vi "AddDropletDBtoDBarrayAndDisplayInGraph.vi"(8 "error in (no error)":errorcluster, 11 "Queue In":refnum<queue>) -> (0 "error out":errorcluster, 3 "Queue Out":refnum<queue>)   [LabVIEW 2013]
doc: "Use this template to build a VI to use as a subVI."
uses:
  TypeDef/DisplayQueue.ctl
  TypeDef/DisplayEnum.ctl
  DB/DbEnum.ctl
  DB/ArrayofDropletsDBEnum.ctl
panel:
  # "Add droplet database to database array\nand update the normalized droplet graph \nas a function of temperature"
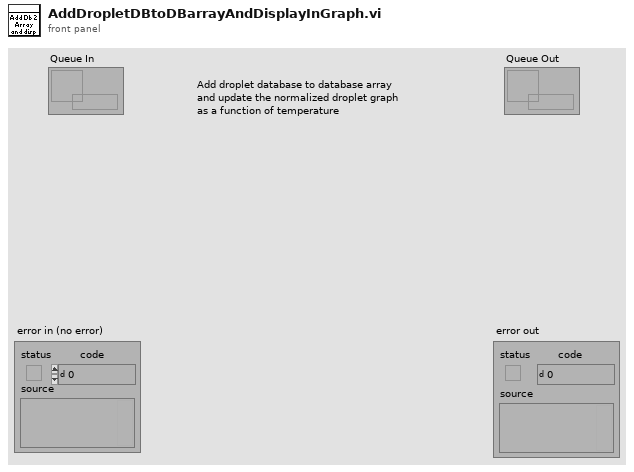
[diagram p1: front panel]
types:
  T1 = typedef "ArrayofDropletsDBEnum.ctl" = enum16{"AnalyzeDropletDBs", "PrepareDBforSave", "GetDBtoListBox", "UpdateDBtoListBox", "AddDBtoListBox", "AddDropletDB", "InitArrayOfDropletDB"}
  T2 = typedef "DisplayEnum.ctl" = enum16{"Stop Display", "Update Display", "Update Multiple Files Display", "Center Image", "Update Configuration Display", "Init Display"}
  T3 = typedef "DbEnum.ctl" = enum16{"RemoveOneDroplet", "AddOneDroplet", "Write DropletDB", "Init", "Insert Detection Result Data", "Insert Grey Level Result", "Insert Baseline Results", "AddFreezeImagesAtCertainDroplet", "UpdateIncludeDroplet", "Insert Freeze Analysis Results", "GetDropDB", "GetNoFreezedDroplets", "GetGreyLevelAndDiff", "GetGreyLevelatIndexTime", "GetDropletsBoundingBox", "GetDropletsDiameter"}
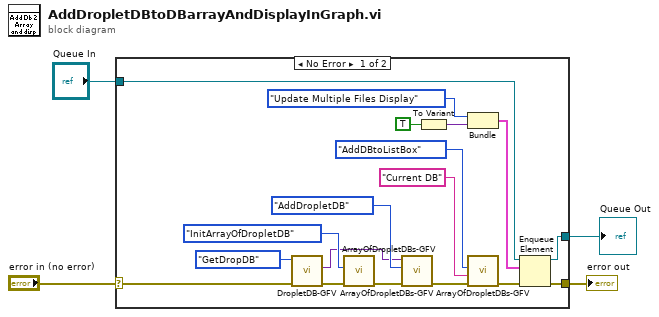
[diagram p0: block diagram]
diagram:
  n1 = case shown="No Error" "error in (no error)" {
    selector: "error in (no error)" -> [w7 w24]
    tunnel: [w6 w24] -> w3
    tunnel: "Queue In" -> [w22 w23]
    tunnel: [w5 w23] -> w1
    frame No Error {
      n2 = call "DropletDB-GFV.vi"("error in (no error)"=w7, "Command In"=DbEnum."GetDropDB") -> ("error out"=w19:errorcluster, "Data out"=w16:variant)  [unwired: 8 in]
      n3 = call "ArrayOfDropletDBs-GFV.vi"("error in (no error)"=w19, 10:ArrayofDropletsDBEnum."InitArrayOfDropletDB") -> ("error out"=w18:errorcluster)  [unwired: 8 in, 1 out]
      n4 = call "ArrayOfDropletDBs-GFV.vi"("error in (no error)"=w18, 10:ArrayofDropletsDBEnum."AddDropletDB", "Data in"=w16) -> ("error out"=w10:errorcluster)  [unwired: 7 in, 1 out]
      n5 = To Variant(anything=TRUE) -> (Variant=w15:variant)
      n6 = Bundle("Enum"=DisplayEnum."Update Multiple Files Display", "Variant"=w15) -> (w12:cluster{"Enum":T2, "Variant":variant})  [unwired: 1 in]
      n7 = call "ArrayOfDropletDBs-GFV.vi"("error in (no error)"=w10, "DB Name"="Current DB", 10:ArrayofDropletsDBEnum."AddDBtoListBox") -> ("error out"=w9:errorcluster)  [unwired: 7 in, 1 out]
      n8 = Enqueue Element(queue=w22, element=w12, error in (no error)=w9) -> (queue out=w5:refnum<queue>, error out=w6:errorcluster)  [unwired: 1 in, 1 out]
    }
    frame Error {
    }
  }
  "error out" <- w3
  "Queue Out" <- w1
